vi "Drive Deadband.vi"(8 "Tank":dbl, 9 "Rotate":dbl, 10 "Forward":dbl, 11 "Translate":dbl) -> (0 "Tank":dbl, 1 "Rotate":dbl, 2 "Forward":dbl, 3 "Translate":dbl)   [LabVIEW 2014]
uses:
  Events.vi
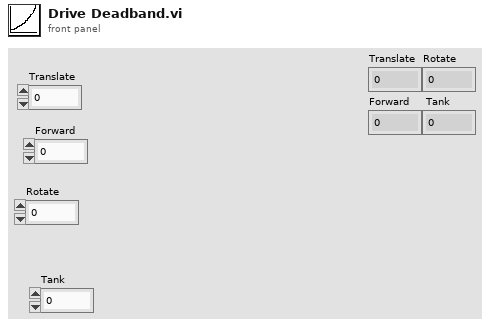
[diagram p1: front panel]
types:
  T1 = cluster{"Shooter latch power":dbl, "Shooter winch power":dbl, "Shooter gearbox servo angles disengaged":i32, "Shooter gearbox servo angles engaged":i32, "Shooter winch power while stalling":dbl, "Exponential Drive Exponent":dbl}
  T2 = cluster{"Translate":dbl, "Y-Axis (Backward Speed)":dbl, "Rotate":dbl, "Tank right side":dbl, "axis 5":dbl, "axis 6":dbl, "Use gyro":bool, "Exponential\ndrive":bool, "Ring light":bool, "PID rotation":bool, "PID Gain":dbl}
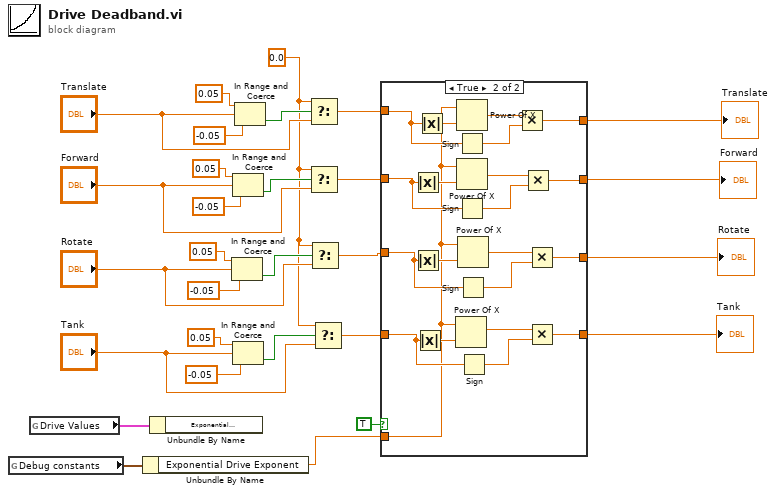
[diagram p0: block diagram]
diagram:
  w5 = 0.0 ("t")
  n1 = global read "Events.vi" "Debug constants"() -> (w3:T1)
  n2 = global read "Events.vi" "Drive Values"() -> (w9:T2)
  n3 = Unbundle By Name(w3) -> ("Exponential Drive Exponent"=w2:dbl)
  n4 = Unbundle By Name(w9) -> ()  [unwired: 1 out]
  n5 = In Range and Coerce(upper limit=0.05, x="Rotate", lower limit=-0.05) -> (In Range?=w24:bool)  [unwired: 1 out]
  n6 = In Range and Coerce(upper limit=0.05, x="Forward", lower limit=-0.05) -> (In Range?=w21:bool)  [unwired: 1 out]
  n7 = In Range and Coerce(upper limit=0.05, x="Tank", lower limit=-0.05) -> (In Range?=w4:bool)  [unwired: 1 out]
  n8 = In Range and Coerce(upper limit=0.05, x="Translate", lower limit=-0.05) -> (In Range?=w18:bool)  [unwired: 1 out]
  n9 = Select(t=w5, s=w18, f="Translate") -> (s? t:f=w16:dbl)
  n10 = Select(t=w5, s=w21, f="Forward") -> (s? t:f=w14:dbl)
  n11 = Select(t=w5, s=w24, f="Rotate") -> (s? t:f=w12:dbl)
  n12 = Select(t=w5, s=w4, f="Tank") -> (s? t:f=w10:dbl)
  n13 = case shown="True" TRUE {
    tunnel: [w33 w53] -> w17
    tunnel: w16 -> [w33 w39]
    tunnel: [w32 w49] -> w15
    tunnel: w14 -> [w32 w42]
    tunnel: [w31 w50] -> w13
    tunnel: w12 -> [w31 w44]
    tunnel: [w30 w51] -> w11
    tunnel: w10 -> [w30 w48]
    tunnel: w2 -> [_ w34]
    frame False {
    }
    frame True {
      n14 = Absolute Value(x=w42) -> (abs(x)=w37:dbl)
      n15 = Absolute Value(x=w44) -> (abs(x)=w36:dbl)
      n16 = Absolute Value(x=w48) -> (abs(x)=w35:dbl)
      n17 = Absolute Value(x=w39) -> (abs(x)=w38:dbl)
      n18 = Power Of X(1:w35, 2:w34) -> (0:w45:dbl)
      n19 = Power Of X(1:w38, 2:w34) -> (0:w40:dbl)
      n20 = Sign(1:w39) -> (0:w54:dbl)
      n21 = Power Of X(1:w37, 2:w34) -> (0:w43:dbl)
      n22 = Sign(1:w42) -> (0:w41:dbl)
      n23 = Power Of X(1:w36, 2:w34) -> (0:w46:dbl)
      n24 = Sign(1:w44) -> (0:w52:dbl)
      n25 = Sign(1:w48) -> (0:w47:dbl)
      n26 = Multiply(x=w40, y=w54) -> (x*y=w53:dbl)
      n27 = Multiply(x=w43, y=w41) -> (x*y=w49:dbl)
      n28 = Multiply(x=w46, y=w52) -> (x*y=w50:dbl)
      n29 = Multiply(x=w45, y=w47) -> (x*y=w51:dbl)
    }
  }
  "Translate" <- w17
  "Forward" <- w15
  "Rotate" <- w13
  "Tank" <- w11
